vi "Check Connection.vi"() -> (2 "pas sv":refnum<k21>, 3 "user quit?":bool)   [LabVIEW 2012]
uses:
  <vilib>/event_ctls.llb/eventvkey.ctl
panel:
  in  "Msg":string="Attempting to Connect..."
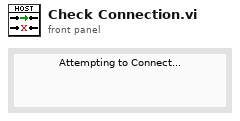
[diagram p1: front panel]
types:
  T1 = enum8{"Enabled", "Disabled", "Disabled and Grayed Out"}
  T2 = cluster{"Read Access":enum8{"Allowed", "Required", "None"}, "Write Access":enum8{"Allowed", "Required", "None"}}
  T3 = typedef "eventvkey.ctl" = enum16{"ASCII", "Enter", "Return", "Shift", "Ctrl", "Alt", "Cmd", "Opt", "Caps", "NumLock", "Clear", "Break", "Up", "Down", "Left", "Right", "Insert", "Delete", "Home", "End", "PageUp", "PageDown", "Escape", "Help", "Pause", "ScrollLock", "F1", "F2", "F3", "F4", "F5", "F6", "F7", "F8", "F9", "F10", "F11", "F12", "F13", "F14", "F15", "F16", "F17", "F18", "F19", "F20", "F21", "F22", "F23", "F24", "Play", "VolumeUp", "VolumeDown", "Mute", "Two Byte Char"}
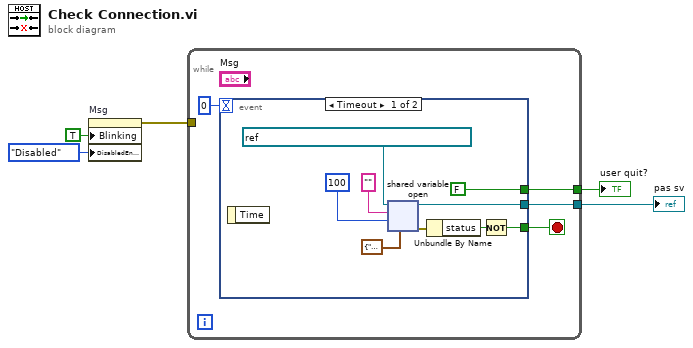
[diagram p0: block diagram]
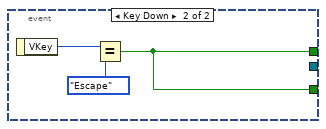
[diagram p2: hidden frame]
diagram:
  n1 = property on="Msg" class="Str"("Blinking"=TRUE, "DisabledEnum"=T1."Disabled" ("Disabled")) -> (error out=w4:errorcluster)  [unwired: 2 in, 1 out]
  n2 = while {
    tunnel: w4 -> [_]
    tunnel: [w8] -> w2
    tunnel: [w6] -> w1
    stop <- w9 stop-if-true
    n3 = event shown="[0] Timeout" {
      selector: _ -> [_ _]
      dyn-events: _ -> [_ _]
      timeout: 0 -> [_ _]
      tunnel: [w10 w19] -> w9
      tunnel: [FALSE w19] -> w8
      tunnel: [w14 _] -> w6
      event Timeout {
        n4 = event-data() -> ()  [unwired: 1 in, 1 out]
        n5 = shared-variable-open(refnum<k21> "ni.var.psp://rt pxi target/PAS_Var/Data" ("shared variable refnum in"), "", T2 {"Read Access"=enum."Required", "Write Access"=enum."None"} ("access"), 100 ("timeout ms")) -> (w14:refnum<k21>, w12:errorcluster)  [unwired: 2 in]
        n6 = Unbundle By Name(w12) -> ("status"=w11:bool)
        n7 = Not(x=w11) -> (.not. x?=w10:bool)
      }
      event Key Down {
        n8 = event-data() -> ("VKey"=w21:T3)  [unwired: 1 in]
        n9 = Equal?(x=w21, y=eventvkey."Escape") -> (x = y?=w19:bool)
      }
    }
  }
  "user quit?" <- w2
  "pas sv" <- w1
